vi "Read Force Demand.vi"(11 "SystemController in":refnum<class "SystemController.lvclass">) -> (2 "Force Demand":T1 format="%.1f", 3 "SystemController out":refnum<class "SystemController.lvclass">)   [LabVIEW 2013]
uses:
  SystemController.lvclass
  Typedefs/ForceDemand.ctl
  Typedefs/M2AADTTypedefs.lvlib
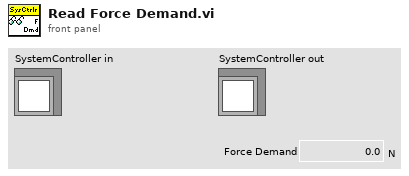
[diagram p1: front panel]
types:
  T1 = typedef "M2AADTTypedefs.lvlib/ForceDemand.ctl" = dbl[unit]
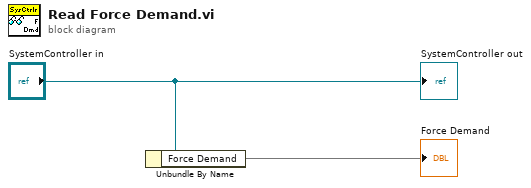
[diagram p0: block diagram]
diagram:
  n1 = Unbundle By Name("SystemController in") -> ("Force Demand"=→"Force Demand")
  "SystemController out" <- "SystemController in"
